vi "Phonendoscope (1).vi"() -> ()   [LabVIEW 2016]
doc: "PHONENDOSCOPE"
uses:
  <vilib>/Analysis/1siggen.llb/Ramp Pattern by Samples.vi
  <vilib>/express/express analysis/Spectral/Block/exnSpectralBlock spectral measurements power poly.vi
  <vilib>/express/express analysis/Spectral/Block/exnSpectralBlock spectral measurements power array WFM.vi
  <vilib>/addons/_NISVFA/_Baseband FFT/SVFA Power Spectrum (N Ch).vi
  <vilib>/express/express analysis/Spectral/Block/exnSpectralBlock spectral measurements power DDT.vi
  <vilib>/express/express analysis/Spectral/XNode/ExpressSpectralMeasurementsBlockNode.xnode
  <vilib>/Analysis/NI_AALPro.lvlib
  <vilib>/Analysis/NI_AAL_SigProc.lvlib
  <vilib>/Analysis/NI_AALBase.lvlib
panel:
  in  "Tab Control":T1(tab)
  out "Найдено":i32=4
  out "Время":dbl[](array[numeric])
  out "Амплитуда":dbl[](array[numeric])
  out "Входной сигнал":cluster{"Locations":dbl[], "Amplitudes":dbl[]}[](graph)
  in  "Порог":dbl(slide) scale=-2.2..2.2
  in  "Макс./Мин.":enum32{"Peaks", "Valleys"}(ring)
  out "AUDIO IN":bool
  out "FILE":bool
  in  "Перключение чтение с файла/myDAQ":bool
  in  "Чтение аудио файла":path
  out "3":bool
  out "2":bool
  in  "Выбор фильтра":i8(slide) scale=0.0..4.0
  out "1":bool
  out "Сигнал на звуковом выходе myDAQ \n(AUDIO OUT)":dynamicdata(graph)
  out "Преобразование Гильберта входного сигнала":dbl[](graph)
  out "Вход.\nсигнал":bool
  out "4":bool
  in  "ВКЛ/ВЫКЛ запись 2":bool
  in  "Запись аудио файла":path
  out "Найдено":i32=4
  out "Время":dbl[](array[numeric])
  out "Амплитуда":dbl[](array[numeric])
  out "Сигнал на выходе фильтра 1":cluster{"Locations":dbl[], "Amplitudes":dbl[]}[](graph)
  in  "Порог":dbl(slide) scale=-2.0..2.0
  in  "Макс./Мин.":enum32{"Peaks", "Valleys"}(ring)
  out "Преобразование Гильберта сигнала на выходе фильтра 1":dbl[](graph)
  out "Найдено":i32=4
  out "Время":dbl[](array[numeric])
  out "Амплитуда":dbl[](array[numeric])
  out "Сигнал на выходе фильтра 2":cluster{"Locations":dbl[], "Amplitudes":dbl[]}[](graph)
  in  "Порог":dbl(slide) scale=-2.0..2.0
  in  "Макс./Мин.":enum32{"Peaks", "Valleys"}(ring)
  out "Преобразование Гильберта сигнала на выходе фильтра 2":dbl[](graph)
  out "Найдено":i32=4
  out "Время":dbl[](array[numeric])
  out "Амплитуда":dbl[](array[numeric])
  out "Сигнал на выходе фильтра 3":cluster{"Locations":dbl[], "Amplitudes":dbl[]}[](graph)
  in  "Порог":dbl(slide) scale=-2.0..2.0
  in  "Макс./Мин.":enum32{"Peaks", "Valleys"}(ring)
  out "Преобразование Гильберта сигнала на выходе фильтра 3":dbl[](graph)
  out "Сигнал на выходе фильтра 4":cluster{"Locations":dbl[], "Amplitudes":dbl[]}[](graph)
  out "Преобразование Гильберта сигнала на выходе фильтра 4":dbl[](graph)
  out "Найдено":i32=4
  out "Время":dbl[](array[numeric])
  out "Амплитуда":dbl[](array[numeric])
  in  "Порог":dbl(slide) scale=-2.0..2.0
  in  "Макс./Мин.":enum32{"Peaks", "Valleys"}(ring)
  out "Спектральная мощность сигнала на входе":cluster{"f0":dbl, "df":dbl, "magnitude":dbl[]}[](graph)
  out "АЧХ на входе":cluster{"f0":dbl, "df":dbl, "magnitude":dbl[]}[](graph)
  out "Спектральная мощность сигнала на выходе фильтра 3":cluster{"f0":dbl, "df":dbl, "magnitude":dbl[]}[](graph)
  out "АЧХ на выходе фильтра 3":dynamicdata(graph)
  out "Спектральная мощность сигнала на выходе фильтра 2":cluster{"f0":dbl, "df":dbl, "magnitude":dbl[]}[](graph)
  out "АЧХ на выходе фильтра 2":dynamicdata(graph)
  out "Спектральная мощность сигнала на выходе фильтра 1":cluster{"f0":dbl, "df":dbl, "magnitude":dbl[]}[](graph)
  out "АЧХ на выходе фильтра 1":dynamicdata(graph)
  out "АЧХ на выходе фильтра 4":dynamicdata(graph)
  out "Спектральная мощность сигнала на выходе фильтра 4":cluster{"f0":dbl, "df":dbl, "magnitude":dbl[]}[](graph)
  # "Виртуальная лаборатория для акустического анализа биомедицинских сигналов с электронного фонендоскопа"
  # "l"
  # "O"
  # "Управление звуковым выходом \nmyDAQ (AUDIO OUT)"
  # "Выбор фильтра"
  # "l"
  # "O"
  # "Частота звука сердечных сокращений (20 Гц - 100 Гц)"
  # "Везикулярное дыхание (18 Гц - 360 Гц)"
  # "Пуэриальное дыхание (400 Гц - 600 Гц)"
  # "Бронхиальное дыхание (700 Гц - 1400 Гц)"
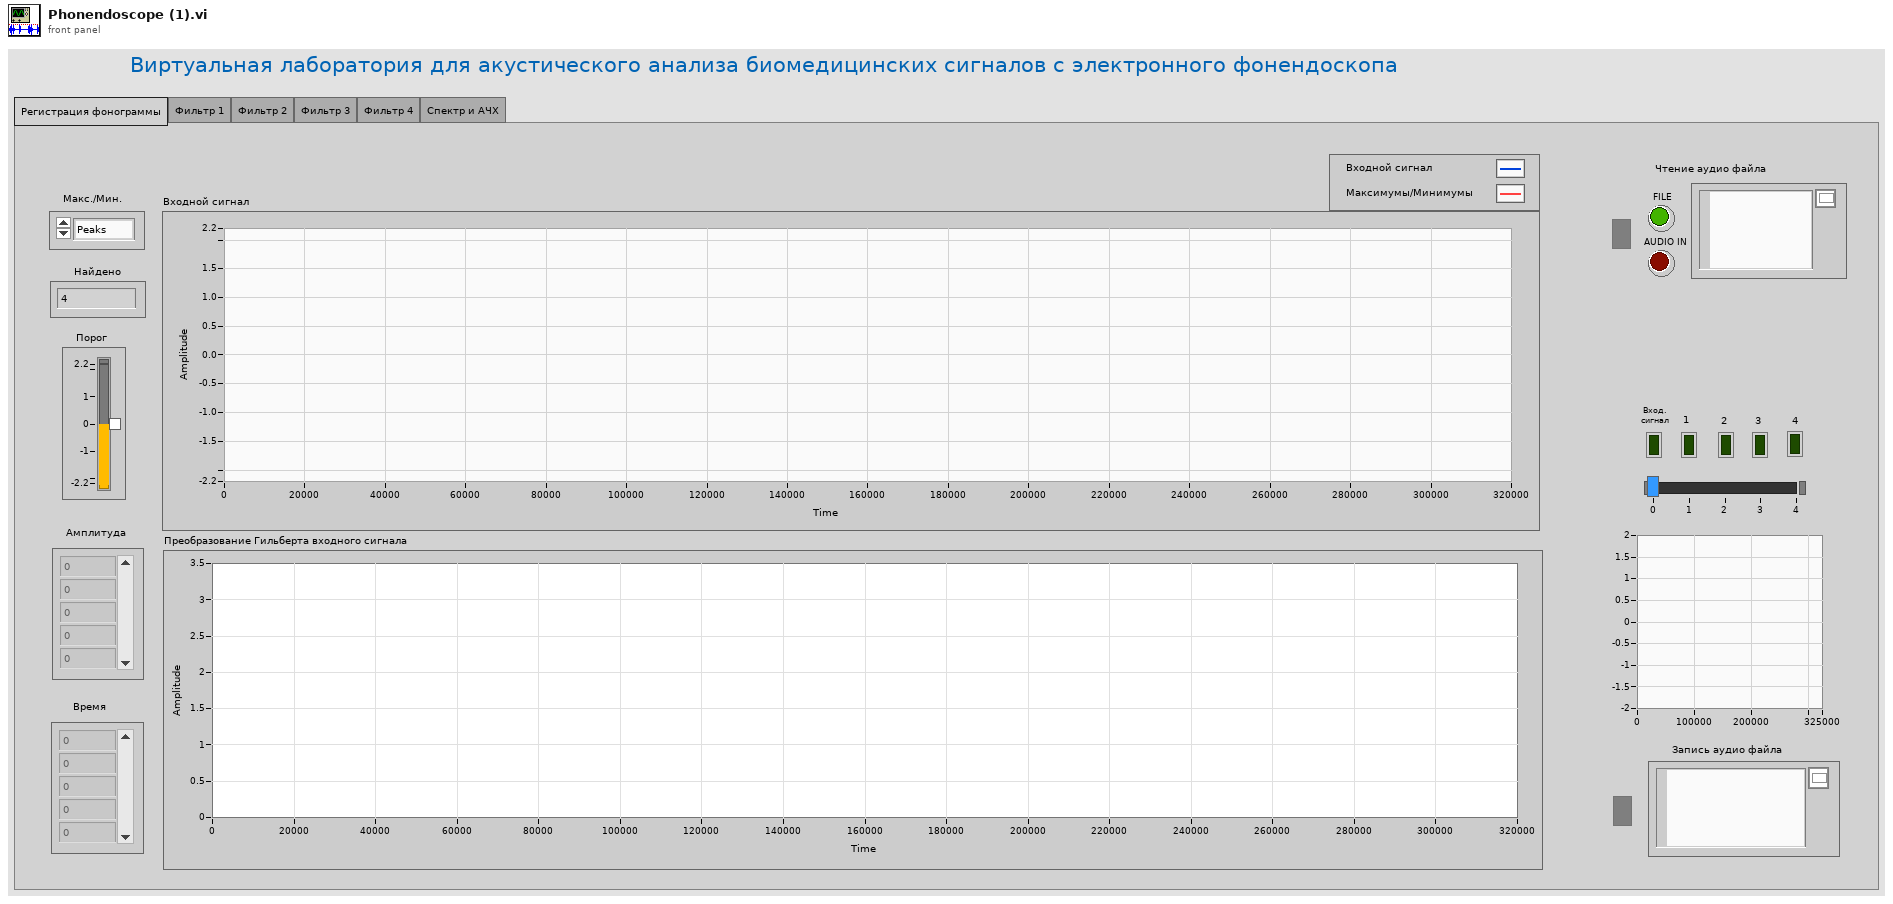
[diagram p1: front panel]
types:
  T1 = enum32{"Регистрация фонограммы", "Фильтр 1", "Фильтр 2", "Фильтр 3", "Фильтр 4", "Спектр и АЧХ"}
  T2 = cluster{"averaging mode":u16, "weighting mode":u16, "number of averages":u32}
  T3 = cluster{"dB On (F)":bool, "unwrap phase (F)":bool, "convert to degree (F)":bool}
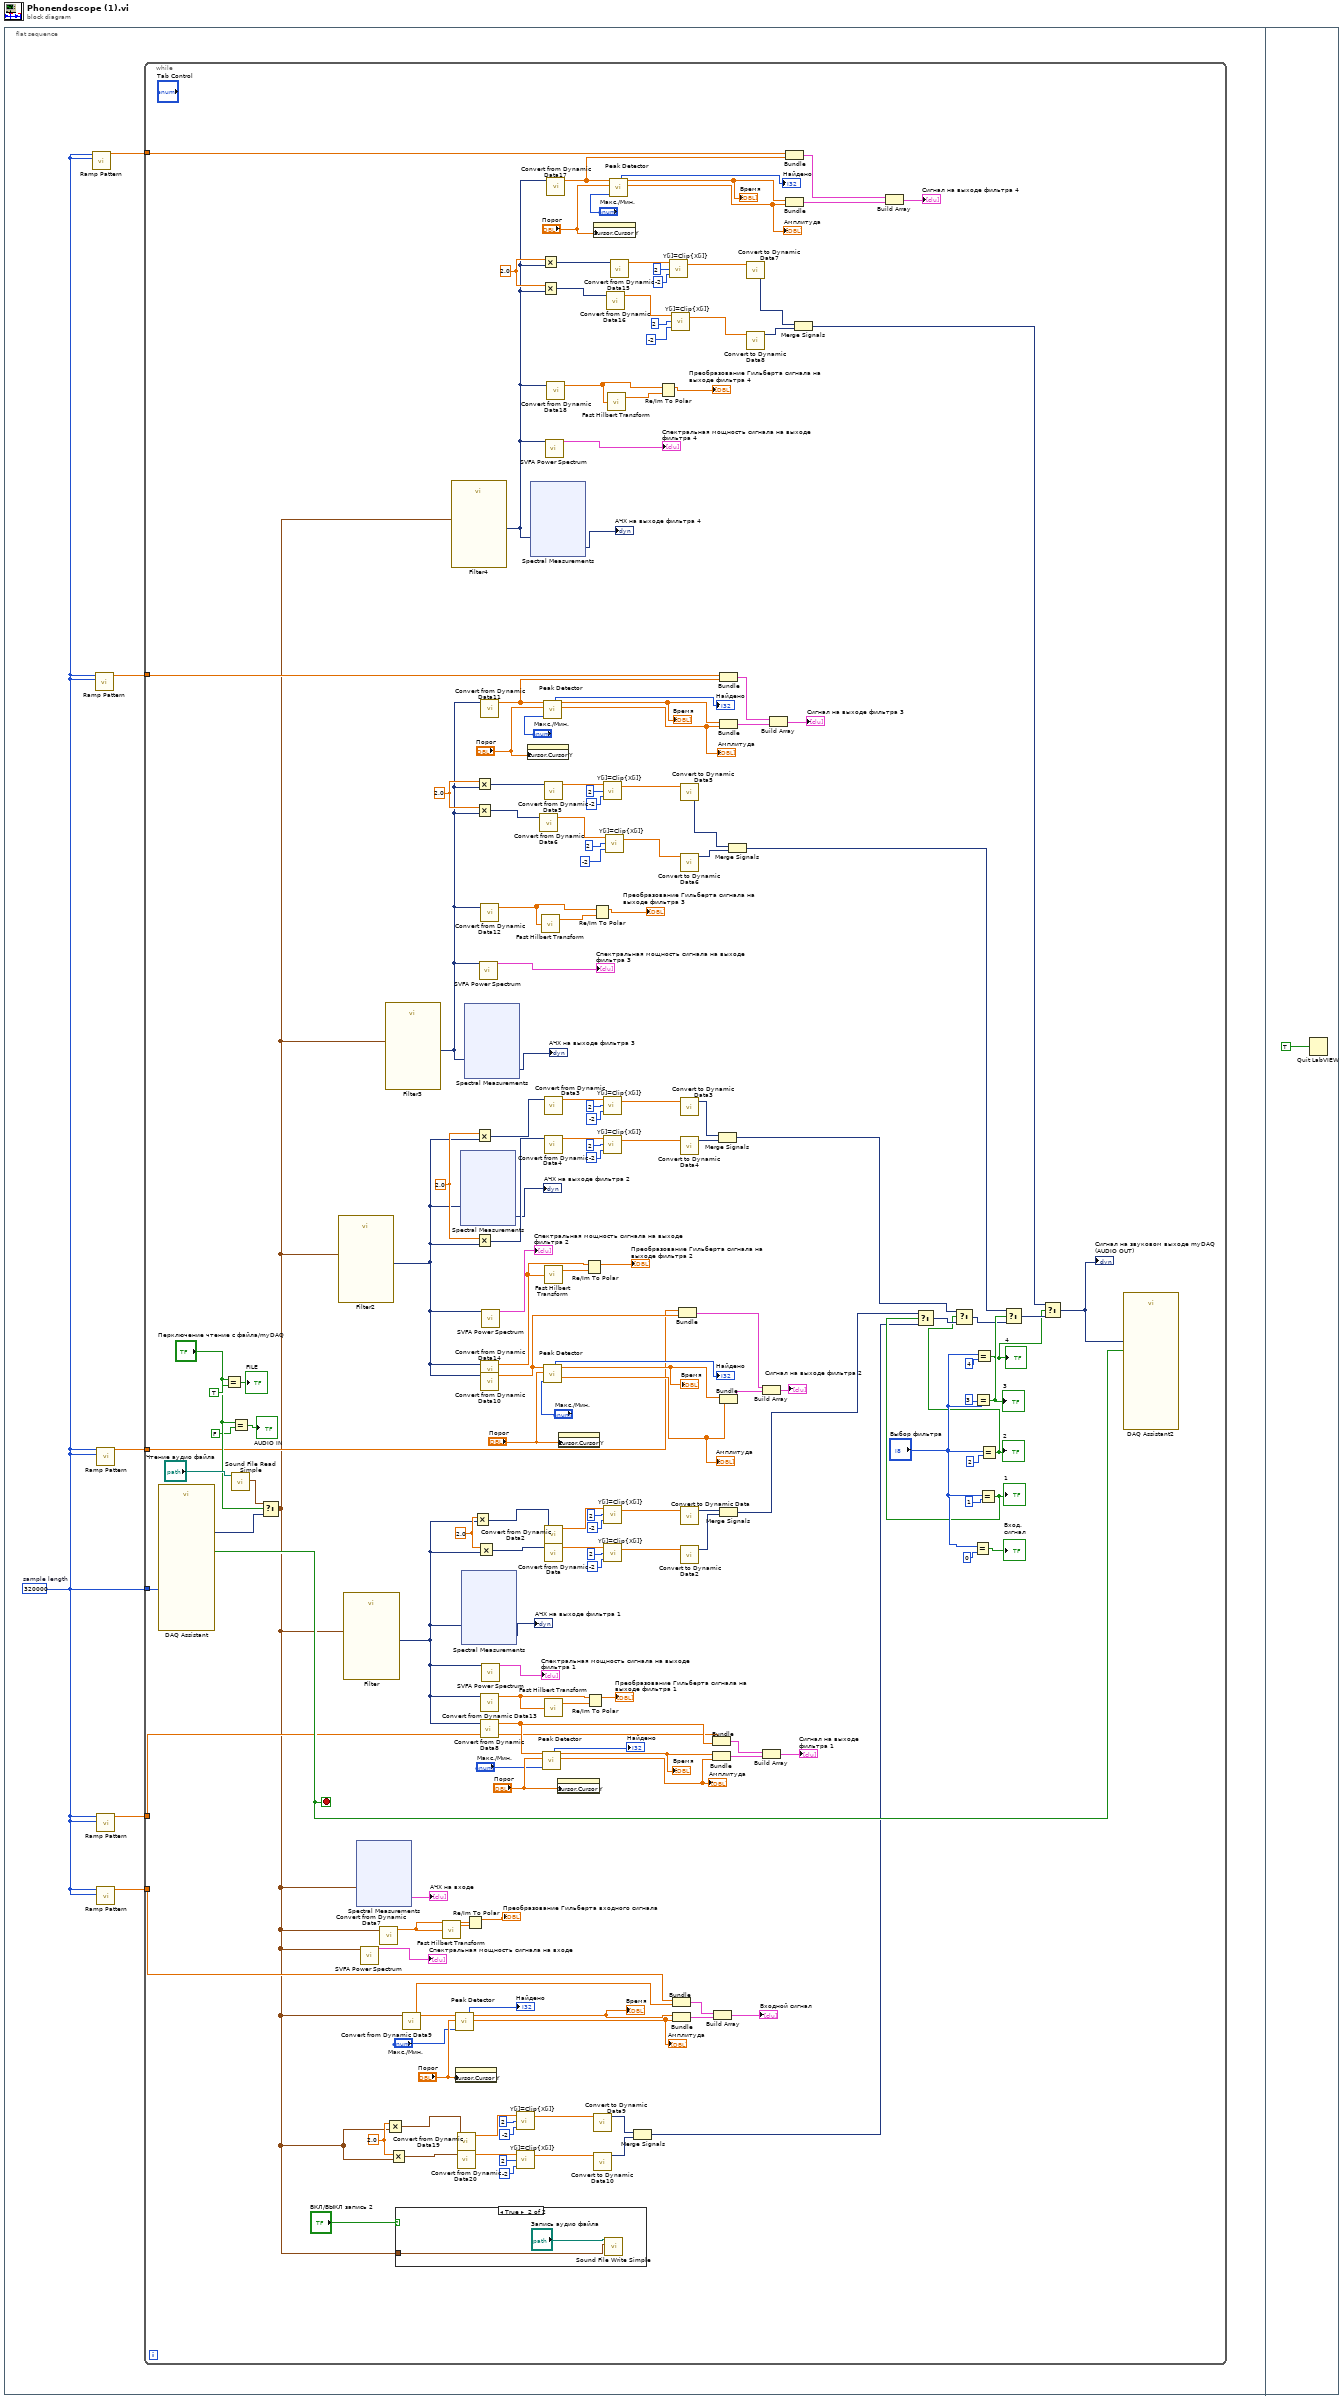
[diagram p0: block diagram]
diagram:
  n1 = flat-sequence {
    frame #0 {
      w2 = 320000  # sample length
      n2 = call-poly <vilib>:"Ramp Pattern.vi"("end"=w2, "samples"=w2) -> ("Ramp Pattern"=w1:dbl[])  [unwired: 8 in, 1 out]
      n3 = call-poly <vilib>:"Ramp Pattern.vi"("end"=w2, "samples"=w2) -> ("Ramp Pattern"=w3:dbl[])  [unwired: 8 in, 1 out]
      n4 = call-poly <vilib>:"Ramp Pattern.vi"("end"=w2, "samples"=w2) -> ("Ramp Pattern"=w4:dbl[])  [unwired: 8 in, 1 out]
      n5 = call-poly <vilib>:"Ramp Pattern.vi"("end"=w2, "samples"=w2) -> ("Ramp Pattern"=w6:dbl[])  [unwired: 8 in, 1 out]
      n6 = call-poly <vilib>:"Ramp Pattern.vi"("end"=w2, "samples"=w2) -> ("Ramp Pattern"=w5:dbl[])  [unwired: 8 in, 1 out]
      n7 = while {
        tunnel: w2 -> [w119]
        tunnel: w6 -> [w118]
        tunnel: w5 -> [w108]
        tunnel: w4 -> [w98]
        tunnel: w3 -> [w88]
        tunnel: w1 -> [w36]
        stop <- w120 stop-if-true
        w21 = 2.0
        w64 = 2.0
        w152 = 2.0
        w168 = 2.0
        w181 = 2.0
        n8 = call "DAQ Assistant"("number of samples"=w119) -> ("data"=w136:dynamicdata, "stopped"=w120:bool)  [unwired: 15 in, 2 out]
        n9 = Equal?(x="Перключение чтение с файла/myDAQ", y=TRUE) -> (x = y?=→"FILE":bool)
        n10 = Equal?(x="Перключение чтение с файла/myDAQ", y=FALSE) -> (x = y?=→"AUDIO IN":bool)
        n11 = call <vilib>:"Sound File Read Simple.vi"("path"="Чтение аудио файла") -> ("data"=w135:waveform(dbl)[])  [unwired: 7 in, 3 out]
        n12 = Select(t=w135, s="Перключение чтение с файла/myDAQ", f=w136) -> (s? t:f=w8:waveform(dbl)[])
        n13 = call "Filter2"("Signal"=w8) -> ("Filtered Signal"=w66:dynamicdata)  [unwired: 9 in, 1 out]
        n14 = call "Filter"("Signal"=w8) -> ("Filtered Signal"=w77:dynamicdata)  [unwired: 9 in, 1 out]
        n15 = xnode "Spectral Measurements"("Signals"=w8) -> ("Power Spectrum"=→"АЧХ на входе":cluster{"f0":dbl, "df":dbl, "magnitude":dbl[]}[])  [unwired: 1 in, 1 out]
        n16 = call-poly <vilib>:"SVFA Power Spectrum.vi"("scaled signals [EU]"=w8) -> ("power spectra [dB EU]"=→"Спектральная мощность сигнала на входе":cluster{"f0":dbl, "df":dbl, "magnitude":dbl[]}[])  [unwired: 13 in, 5 out]
        n17 = call "Convert from Dynamic Data7"("Dynamic Data Type"=w8) -> ("Array"=w74:dbl[])  [unwired: 3 in]
        n18 = call "Filter3"("Signal"=w8) -> ("Filtered Signal"=w70:dynamicdata)  [unwired: 9 in, 1 out]
        n19 = Multiply(x=w21, y=w8) -> (x*y=w18:waveform(dbl)[])
        n20 = Multiply(x=w21, y=w8) -> (x*y=w12:waveform(dbl)[])
        n21 = case shown="True" "ВКЛ/ВЫКЛ запись 2" {
          tunnel: w8 -> [_ w192]
          frame False {
          }
          frame True {
            n22 = call <vilib>:"Sound File Write Simple.vi"("data"=w192, "path"="Запись аудио файла") -> ()  [unwired: 8 in, 2 out]
          }
        }
        n23 = call "Convert from Dynamic Data9"("Dynamic Data Type"=w8) -> ("Array"=w110:dbl[])  [unwired: 3 in]
        n24 = call <vilib>:"Fast Hilbert Transform.vi"("X"=w74) -> ("Hilbert{X}"=w75:dbl[])  [unwired: 1 out]
        n25 = call "Filter4"("Signal"=w8) -> ("Filtered Signal"=w37:dynamicdata)  [unwired: 9 in, 1 out]
        n26 = call <vilib>:"Peak Detector.vi"("peaks/valleys"="Макс./Мин.", "threshold"="Порог", "X"=w110) -> ("Amplitudes"=w113:dbl[], "Locations"=w112:dbl[], "# found"=→"Найдено":i32)  [unwired: 4 in, 2 out]
        "Время" <- w112
        "Амплитуда" <- w113
        n27 = property on="Входной сигнал" class="XYGraph (strict)"("Cursor.Cursor Y"="Порог") -> ()  [unwired: 2 in, 2 out]
        n28 = call "Convert from Dynamic Data19"("Dynamic Data Type"=w18) -> ("Array"=w17:dbl[])  [unwired: 3 in]
        n29 = call "Convert from Dynamic Data20"("Dynamic Data Type"=w12) -> ("Array"=w11:dbl[])  [unwired: 3 in]
        n30 = xnode "Spectral Measurements"("Signals"=w66) -> ("Power Spectrum"=→"АЧХ на выходе фильтра 2":dynamicdata)  [unwired: 1 in, 1 out]
        n31 = xnode "Spectral Measurements"("Signals"=w77) -> ("Power Spectrum"=→"АЧХ на выходе фильтра 1":dynamicdata)  [unwired: 1 in, 1 out]
        n32 = xnode "Spectral Measurements"("Signals"=w70) -> ("Power Spectrum"=→"АЧХ на выходе фильтра 3":dynamicdata)  [unwired: 1 in, 1 out]
        n33 = Re/Im To Polar(2:w75, 3:w74) -> (1:→"Преобразование Гильберта входного сигнала":dbl[])  [unwired: 1 out]
        n34 = Multiply(x=w181, y=w77) -> (x*y=w178:dynamicdata)
        n35 = Multiply(x=w152, y=w70) -> (x*y=w149:dynamicdata)
        n36 = Multiply(x=w152, y=w70) -> (x*y=w143:dynamicdata)
        n37 = Multiply(x=w168, y=w66) -> (x*y=w165:dynamicdata)
        n38 = Multiply(x=w168, y=w66) -> (x*y=w159:dynamicdata)
        n39 = Multiply(x=w181, y=w77) -> (x*y=w172:dynamicdata)
        n40 = call-poly <vilib>:"SVFA Power Spectrum.vi"("scaled signals [EU]"=w70) -> ("power spectra [dB EU]"=→"Спектральная мощность сигнала на выходе фильтра 3":cluster{"f0":dbl, "df":dbl, "magnitude":dbl[]}[])  [unwired: 13 in, 5 out]
        n41 = call "Convert from Dynamic Data8"("Dynamic Data Type"=w77) -> ("Array"=w122:dbl[])  [unwired: 3 in]
        n42 = call "Convert from Dynamic Data11"("Dynamic Data Type"=w70) -> ("Array"=w90:dbl[])  [unwired: 3 in]
        n43 = call "Convert from Dynamic Data12"("Dynamic Data Type"=w70) -> ("Array"=w71:dbl[])  [unwired: 3 in]
        n44 = call "Convert from Dynamic Data14"("Dynamic Data Type"=w66) -> ("Array"=w67:dbl[])  [unwired: 3 in]
        n45 = call "Convert from Dynamic Data10"("Dynamic Data Type"=w66) -> ("Array"=w100:dbl[])  [unwired: 3 in]
        n46 = call "Convert from Dynamic Data13"("Dynamic Data Type"=w77) -> ("Array"=w79:dbl[])  [unwired: 3 in]
        n47 = call-poly <vilib>:"SVFA Power Spectrum.vi"("scaled signals [EU]"=w66) -> ("power spectra [dB EU]"=→"Спектральная мощность сигнала на выходе фильтра 2":cluster{"f0":dbl, "df":dbl, "magnitude":dbl[]}[])  [unwired: 13 in, 5 out]
        n48 = call-poly <vilib>:"SVFA Power Spectrum.vi"("scaled signals [EU]"=w77) -> ("power spectra [dB EU]"=→"Спектральная мощность сигнала на выходе фильтра 1":cluster{"f0":dbl, "df":dbl, "magnitude":dbl[]}[])  [unwired: 13 in, 5 out]
        n49 = call <vilib>:"Y[i]=Clip{X[i]}.vi"("lower limit"=-2, "upper limit"=2, "Input Array"=w17) -> ("Clipped Array"=w16:dbl[])  [unwired: 1 out]
        n50 = call <vilib>:"Y[i]=Clip{X[i]}.vi"("lower limit"=-2, "upper limit"=2, "Input Array"=w11) -> ("Clipped Array"=w10:dbl[])  [unwired: 1 out]
        n51 = property on="Сигнал на выходе фильтра 3" class="XYGraph (strict)"("Cursor.Cursor Y"="Порог") -> ()  [unwired: 2 in, 2 out]
        n52 = xnode "Spectral Measurements"("Signals"=w37) -> ("Power Spectrum"=→"АЧХ на выходе фильтра 4":dynamicdata)  [unwired: 1 in, 1 out]
        n53 = call "Convert from Dynamic Data6"("Dynamic Data Type"=w143) -> ("Array"=w142:dbl[])  [unwired: 3 in]
        n54 = call <vilib>:"Fast Hilbert Transform.vi"("X"=w71) -> ("Hilbert{X}"=w72:dbl[])  [unwired: 1 out]
        n55 = Multiply(x=w64, y=w37) -> (x*y=w61:dynamicdata)
        n56 = Multiply(x=w64, y=w37) -> (x*y=w55:dynamicdata)
        n57 = call <vilib>:"Peak Detector.vi"("peaks/valleys"="Макс./Мин.", "threshold"="Порог", "X"=w122) -> ("Amplitudes"=w125:dbl[], "Locations"=w124:dbl[], "# found"=→"Найдено":i32)  [unwired: 4 in, 2 out]
        "Время" <- w124
        "Амплитуда" <- w125
        n58 = call <vilib>:"Peak Detector.vi"("peaks/valleys"="Макс./Мин.", "threshold"="Порог", "X"=w90) -> ("Amplitudes"=w93:dbl[], "Locations"=w92:dbl[], "# found"=→"Найдено":i32)  [unwired: 4 in, 2 out]
        "Время" <- w92
        "Амплитуда" <- w93
        n59 = call <vilib>:"Peak Detector.vi"("peaks/valleys"="Макс./Мин.", "threshold"="Порог", "X"=w100) -> ("Amplitudes"=w103:dbl[], "Locations"=w102:dbl[], "# found"=→"Найдено":i32)  [unwired: 4 in, 2 out]
        "Время" <- w102
        "Амплитуда" <- w103
        n60 = call "Convert from Dynamic Data5"("Dynamic Data Type"=w149) -> ("Array"=w148:dbl[])  [unwired: 3 in]
        n61 = call "Convert from Dynamic Data3"("Dynamic Data Type"=w165) -> ("Array"=w164:dbl[])  [unwired: 3 in]
        n62 = call "Convert from Dynamic Data4"("Dynamic Data Type"=w159) -> ("Array"=w158:dbl[])  [unwired: 3 in]
        n63 = call <vilib>:"Fast Hilbert Transform.vi"("X"=w67) -> ("Hilbert{X}"=w68:dbl[])  [unwired: 1 out]
        n64 = call "Convert from Dynamic Data2"("Dynamic Data Type"=w178) -> ("Array"=w177:dbl[])  [unwired: 3 in]
        n65 = call "Convert from Dynamic Data"("Dynamic Data Type"=w172) -> ("Array"=w171:dbl[])  [unwired: 3 in]
        n66 = call <vilib>:"Fast Hilbert Transform.vi"("X"=w79) -> ("Hilbert{X}"=w80:dbl[])  [unwired: 1 out]
        n67 = call-poly <vilib>:"SVFA Power Spectrum.vi"("scaled signals [EU]"=w37) -> ("power spectra [dB EU]"=→"Спектральная мощность сигнала на выходе фильтра 4":cluster{"f0":dbl, "df":dbl, "magnitude":dbl[]}[])  [unwired: 13 in, 5 out]
        n68 = call "Convert from Dynamic Data17"("Dynamic Data Type"=w37) -> ("Array"=w44:dbl[])  [unwired: 3 in]
        n69 = call "Convert from Dynamic Data18"("Dynamic Data Type"=w37) -> ("Array"=w38:dbl[])  [unwired: 3 in]
        n70 = property on="Сигнал на выходе фильтра 1" class="XYGraph (strict)"("Cursor.Cursor Y"="Порог") -> ()  [unwired: 2 in, 2 out]
        n71 = property on="Сигнал на выходе фильтра 2" class="XYGraph (strict)"("Cursor.Cursor Y"="Порог") -> ()  [unwired: 2 in, 2 out]
        n72 = Re/Im To Polar(2:w68, 3:w67) -> (1:→"Преобразование Гильберта сигнала на выходе фильтра 2":dbl[])  [unwired: 1 out]
        n73 = Re/Im To Polar(2:w80, 3:w79) -> (1:→"Преобразование Гильберта сигнала на выходе фильтра 1":dbl[])  [unwired: 1 out]
        n74 = Re/Im To Polar(2:w72, 3:w71) -> (1:→"Преобразование Гильберта сигнала на выходе фильтра 3":dbl[])  [unwired: 1 out]
        n75 = call "Convert to Dynamic Data9"("Array"=w16) -> ("Dynamic Data Type"=w15:dynamicdata)  [unwired: 3 in]
        n76 = call "Convert to Dynamic Data10"("Array"=w10) -> ("Dynamic Data Type"=w9:dynamicdata)  [unwired: 3 in]
        n77 = property on="Сигнал на выходе фильтра 4" class="XYGraph (strict)"("Cursor.Cursor Y"="Порог") -> ()  [unwired: 2 in, 2 out]
        n78 = call <vilib>:"Y[i]=Clip{X[i]}.vi"("lower limit"=-2, "upper limit"=2, "Input Array"=w148) -> ("Clipped Array"=w147:dbl[])  [unwired: 1 out]
        n79 = call <vilib>:"Y[i]=Clip{X[i]}.vi"("lower limit"=-2, "upper limit"=2, "Input Array"=w164) -> ("Clipped Array"=w163:dbl[])  [unwired: 1 out]
        n80 = call <vilib>:"Y[i]=Clip{X[i]}.vi"("lower limit"=-2, "upper limit"=2, "Input Array"=w158) -> ("Clipped Array"=w157:dbl[])  [unwired: 1 out]
        n81 = call <vilib>:"Y[i]=Clip{X[i]}.vi"("lower limit"=-2, "upper limit"=2, "Input Array"=w177) -> ("Clipped Array"=w176:dbl[])  [unwired: 1 out]
        n82 = call <vilib>:"Y[i]=Clip{X[i]}.vi"("lower limit"=-2, "upper limit"=2, "Input Array"=w171) -> ("Clipped Array"=w170:dbl[])  [unwired: 1 out]
        n83 = call <vilib>:"Y[i]=Clip{X[i]}.vi"("lower limit"=-2, "upper limit"=2, "Input Array"=w142) -> ("Clipped Array"=w141:dbl[])  [unwired: 1 out]
        n84 = call "Convert from Dynamic Data16"("Dynamic Data Type"=w55) -> ("Array"=w54:dbl[])  [unwired: 3 in]
        n85 = call <vilib>:"Fast Hilbert Transform.vi"("X"=w38) -> ("Hilbert{X}"=w39:dbl[])  [unwired: 1 out]
        n86 = call <vilib>:"Peak Detector.vi"("peaks/valleys"="Макс./Мин.", "threshold"="Порог", "X"=w44) -> ("Amplitudes"=w47:dbl[], "Locations"=w46:dbl[], "# found"=→"Найдено":i32)  [unwired: 4 in, 2 out]
        "Время" <- w46
        "Амплитуда" <- w47
        n87 = call "Convert from Dynamic Data15"("Dynamic Data Type"=w61) -> ("Array"=w60:dbl[])  [unwired: 3 in]
        n88 = Merge Signals(w15, w9) -> (w7:dynamicdata)
        n89 = Re/Im To Polar(2:w39, 3:w38) -> (1:→"Преобразование Гильберта сигнала на выходе фильтра 4":dbl[])  [unwired: 1 out]
        n90 = call <vilib>:"Y[i]=Clip{X[i]}.vi"("lower limit"=-2, "upper limit"=2, "Input Array"=w60) -> ("Clipped Array"=w59:dbl[])  [unwired: 1 out]
        n91 = call <vilib>:"Y[i]=Clip{X[i]}.vi"("lower limit"=-2, "upper limit"=2, "Input Array"=w54) -> ("Clipped Array"=w53:dbl[])  [unwired: 1 out]
        n92 = Bundle("Ramp Pattern"=w108, "Array"=w110) -> (w117:cluster{"Ramp Pattern":dbl[], "Array":dbl[]})  [unwired: 1 out]
        n93 = Bundle("Locations"=w112, "Amplitudes"=w113) -> (w115:cluster{"Locations":dbl[], "Amplitudes":dbl[]})  [unwired: 1 out]
        n94 = Bundle("Ramp Pattern"=w98, "Array"=w100) -> (w107:cluster{"Ramp Pattern":dbl[], "Array":dbl[]})  [unwired: 1 out]
        n95 = call "Convert to Dynamic Data5"("Array"=w147) -> ("Dynamic Data Type"=w146:dynamicdata)  [unwired: 3 in]
        n96 = call "Convert to Dynamic Data6"("Array"=w141) -> ("Dynamic Data Type"=w140:dynamicdata)  [unwired: 3 in]
        n97 = call "Convert to Dynamic Data3"("Array"=w163) -> ("Dynamic Data Type"=w162:dynamicdata)  [unwired: 3 in]
        n98 = call "Convert to Dynamic Data4"("Array"=w157) -> ("Dynamic Data Type"=w156:dynamicdata)  [unwired: 3 in]
        n99 = call "Convert to Dynamic Data"("Array"=w176) -> ("Dynamic Data Type"=w175:dynamicdata)  [unwired: 3 in]
        n100 = call "Convert to Dynamic Data2"("Array"=w170) -> ("Dynamic Data Type"=w169:dynamicdata)  [unwired: 3 in]
        n101 = Bundle("Ramp Pattern"=w118, "Array"=w122) -> (w129:cluster{"Ramp Pattern":dbl[], "Array":dbl[]})  [unwired: 1 out]
        n102 = Bundle("Locations"=w124, "Amplitudes"=w125) -> (w127:cluster{"Locations":dbl[], "Amplitudes":dbl[]})  [unwired: 1 out]
        n103 = Build Array(w117, w115) -> (→"Входной сигнал":cluster{"Locations":dbl[], "Amplitudes":dbl[]}[])
        n104 = Merge Signals(w162, w156) -> (w25:dynamicdata)
        n105 = Merge Signals(w175, w169) -> (w24:dynamicdata)
        n106 = Bundle("Ramp Pattern"=w88, "Array"=w90) -> (w97:cluster{"Ramp Pattern":dbl[], "Array":dbl[]})  [unwired: 1 out]
        n107 = Bundle("Locations"=w92, "Amplitudes"=w93) -> (w95:cluster{"Locations":dbl[], "Amplitudes":dbl[]})  [unwired: 1 out]
        n108 = Bundle("Locations"=w102, "Amplitudes"=w103) -> (w105:cluster{"Locations":dbl[], "Amplitudes":dbl[]})  [unwired: 1 out]
        n109 = Merge Signals(w146, w140) -> (w138:dynamicdata)
        n110 = call "Convert to Dynamic Data7"("Array"=w59) -> ("Dynamic Data Type"=w58:dynamicdata)  [unwired: 3 in]
        n111 = call "Convert to Dynamic Data8"("Array"=w53) -> ("Dynamic Data Type"=w52:dynamicdata)  [unwired: 3 in]
        n112 = Build Array(w107, w105) -> (→"Сигнал на выходе фильтра 2":cluster{"Locations":dbl[], "Amplitudes":dbl[]}[])
        n113 = Build Array(w129, w127) -> (→"Сигнал на выходе фильтра 1":cluster{"Locations":dbl[], "Amplitudes":dbl[]}[])
        n114 = Build Array(w97, w95) -> (→"Сигнал на выходе фильтра 3":cluster{"Locations":dbl[], "Amplitudes":dbl[]}[])
        n115 = Bundle("Ramp Pattern"=w36, "Array"=w44) -> (w51:cluster{"Ramp Pattern":dbl[], "Array":dbl[]})  [unwired: 1 out]
        n116 = Bundle("Locations"=w46, "Amplitudes"=w47) -> (w49:cluster{"Locations":dbl[], "Amplitudes":dbl[]})  [unwired: 1 out]
        n117 = Merge Signals(w58, w52) -> (w35:dynamicdata)
        n118 = Build Array(w51, w49) -> (→"Сигнал на выходе фильтра 4":cluster{"Locations":dbl[], "Amplitudes":dbl[]}[])
        n119 = Equal?(x="Выбор фильтра", y=i8 0) -> (x = y?=→"Вход.\nсигнал":bool)
        n120 = Equal?(x="Выбор фильтра", y=i8 3) -> (x = y?=w139:bool)
        "3" <- w139
        n121 = Equal?(x="Выбор фильтра", y=i8 4) -> (x = y?=w28:bool)
        "4" <- w28
        n122 = Equal?(x="Выбор фильтра", y=i8 1) -> (x = y?=w23:bool)
        "1" <- w23
        n123 = Select(t=w24, s=w23, f=w7) -> (s? t:f=w26:dynamicdata)
        n124 = Equal?(x="Выбор фильтра", y=i8 2) -> (x = y?=w22:bool)
        "2" <- w22
        n125 = Select(t=w25, s=w22, f=w26) -> (s? t:f=w27:dynamicdata)
        n126 = Select(t=w138, s=w139, f=w27) -> (s? t:f=w30:dynamicdata)
        n127 = Select(t=w35, s=w28, f=w30) -> (s? t:f=w31:dynamicdata)
        "Сигнал на звуковом выходе myDAQ \n(AUDIO OUT)" <- w31
        n128 = call "DAQ Assistant2"("data"=w31, "stop (F)"=w120) -> ()  [unwired: 15 in, 3 out]
      }
    }
    frame #1 {
      n129 = Quit LabVIEW(quit? (T)=TRUE) -> ()
    }
  }
